vi "mani.vi"   [LabVIEW 2021]
uses:
  <vilib>/Waveform/DWDTOps.llb/DWDT Analog to Digital.vi
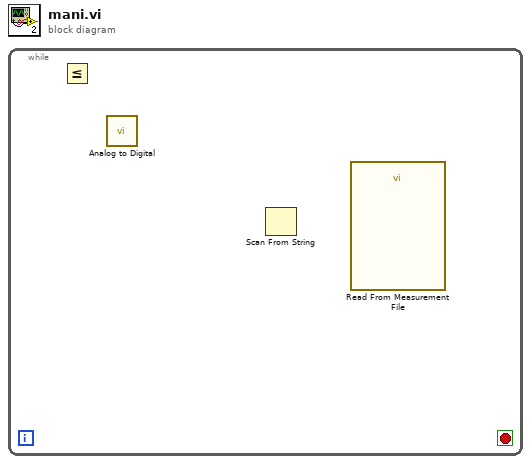
[diagram p0: block diagram]
diagram:
  n1 = while {
    stop <- _ stop-if-true
    n2 = Less Or Equal?() -> ()  [unwired: 2 in, 1 out]
    n3 = call-poly <vilib>:"Analog to Digital.vi"() -> ()  [unwired: 8 in, 4 out]
    n4 = Scan From String() -> ()  [unwired: 5 in, 2 out]
    n5 = call "Read From Measurement File"() -> ()  [unwired: 6 in, 6 out]
  }
